vi "Iso Measurement Read.vi"(8 "error in":errorcluster, 11 "Cycler in":refnum<class "Cycler.lvclass">) -> (0 "error out":errorcluster, 1 "Changed or First Call?":bool, 2 "Iso Measurement ACT":bool, 3 "Cycler out":refnum<class "Cycler.lvclass">)   [LabVIEW 2023, in "Cycler.lvclass"]
uses:
  Cycler.lvclass
  Low Level Capabilities/Iso Measurement/Iso Measurement.lvclass
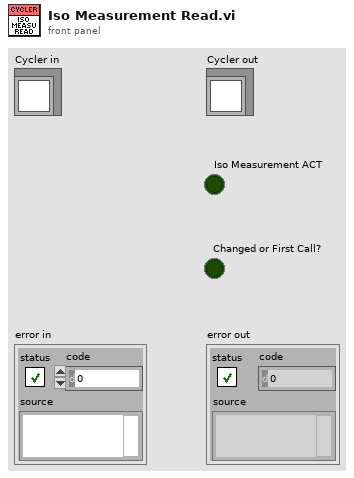
[diagram p1: front panel]
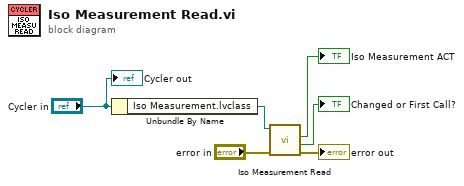
[diagram p0: block diagram]
diagram:
  n1 = Unbundle By Name("Cycler in") -> ("Iso Measurement.lvclass"=w5:refnum<class "Iso Measurement.lvclass">)
  n2 = call-dynamic "Iso Measurement Read.vi"("error in"="error in", "Iso Measurement in"=w5) -> ("error out"=→"error out":errorcluster, "Changed or First Call?"=→"Changed or First Call?":bool, "Iso Measurement ACT"=→"Iso Measurement ACT":bool)  [unwired: 6 in, 1 out]
  "Cycler out" <- "Cycler in"
